vi "Condition _string.vi"(10 "Shift":string(combo)="ALL", 11 "Select Line 2":string(combo)="ST 1") -> (0 "String":string, 2 "condition":string, 3 "x .and. y?":bool)   [LabVIEW 2017]
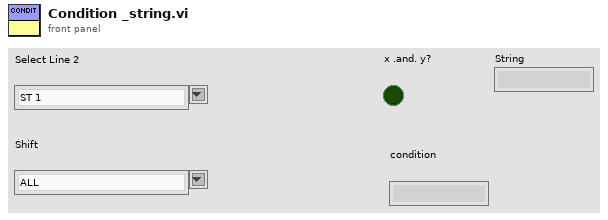
[diagram p1: front panel]
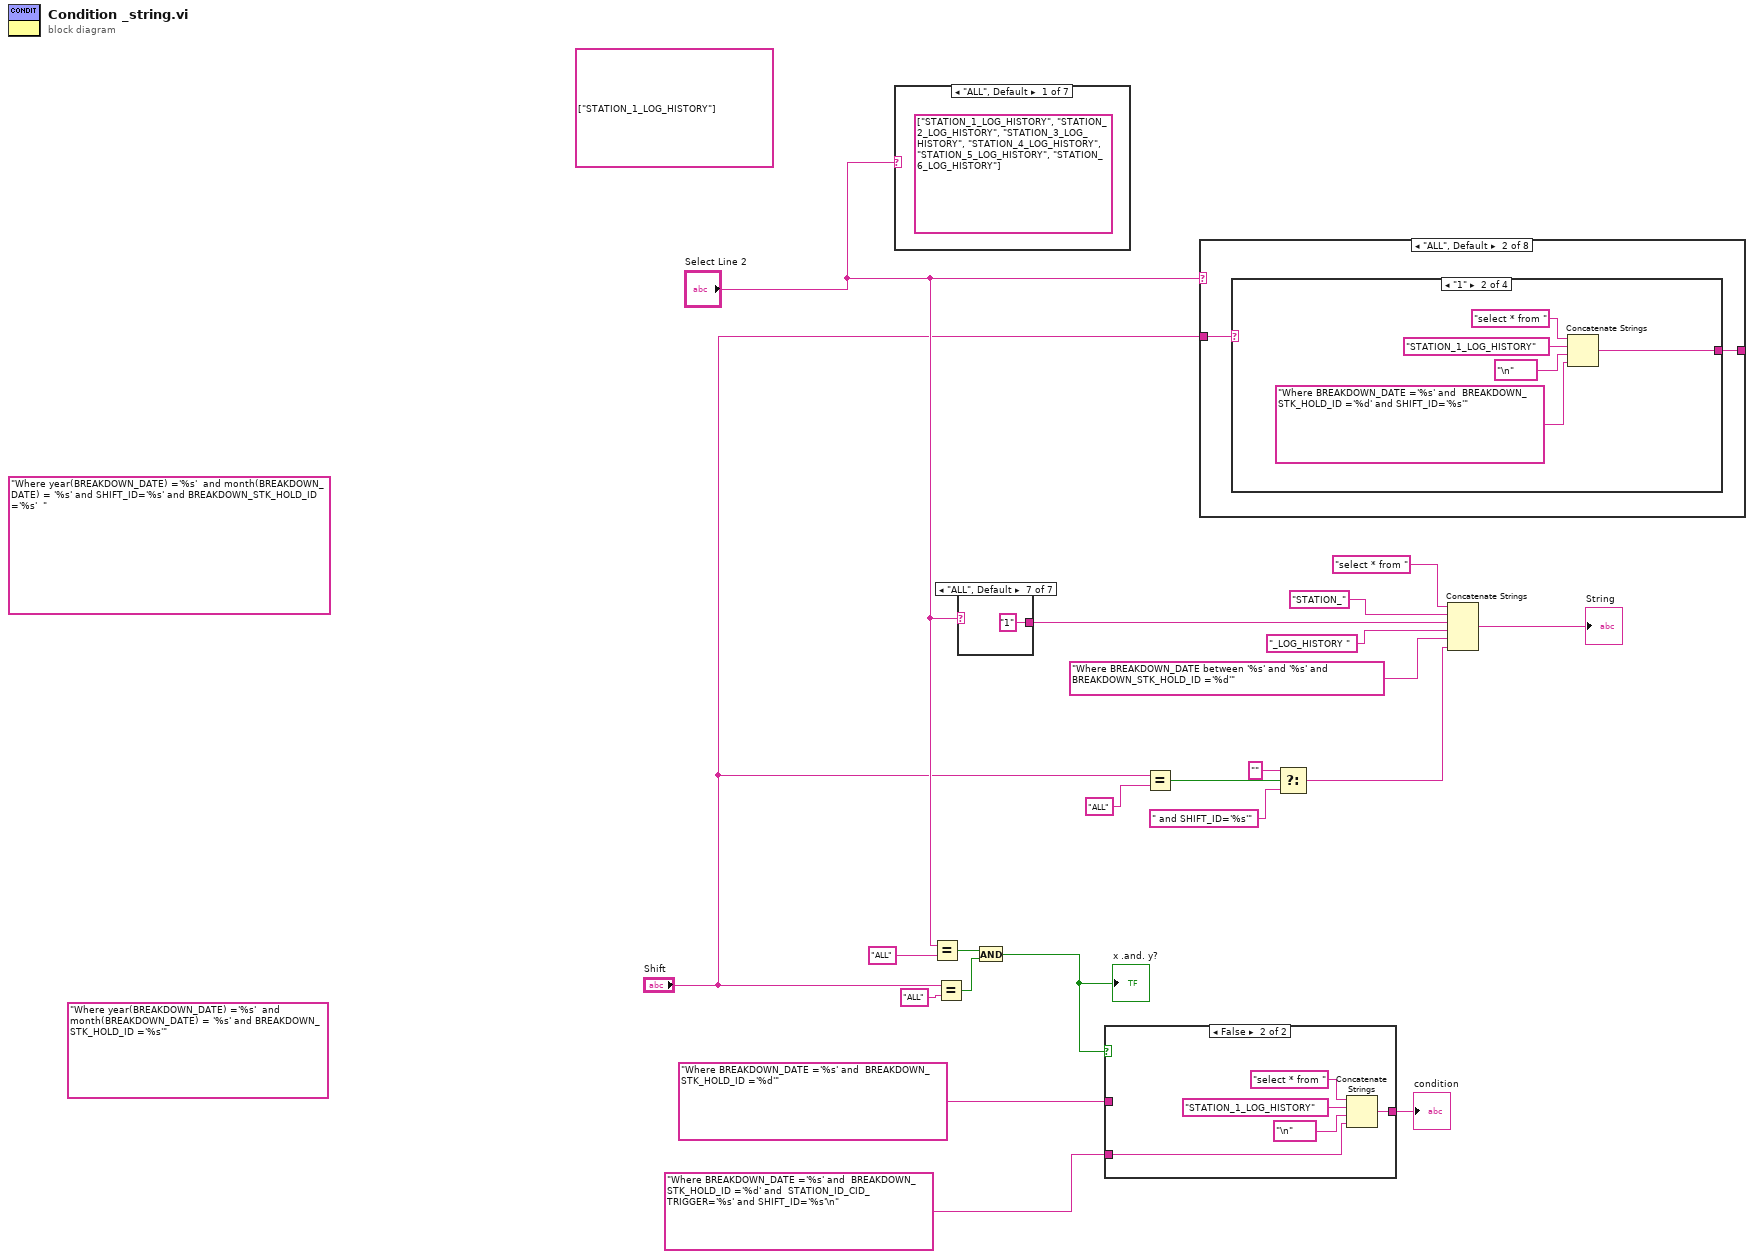
[diagram p0: block diagram]
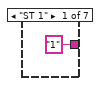
[diagram p2: hidden frame]
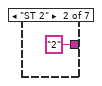
[diagram p3: hidden frame]
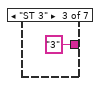
[diagram p4: hidden frame]
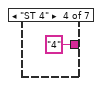
[diagram p5: hidden frame]
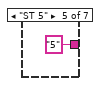
[diagram p6: hidden frame]
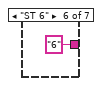
[diagram p7: hidden frame]
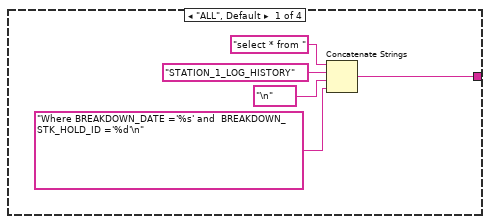
[diagram p9: hidden frame]
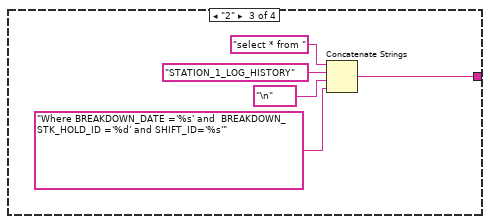
[diagram p10: hidden frame]
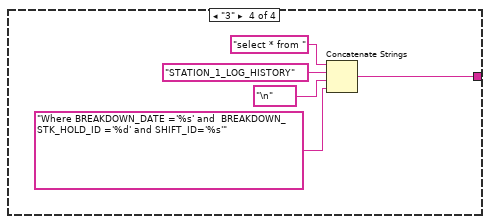
[diagram p11: hidden frame]
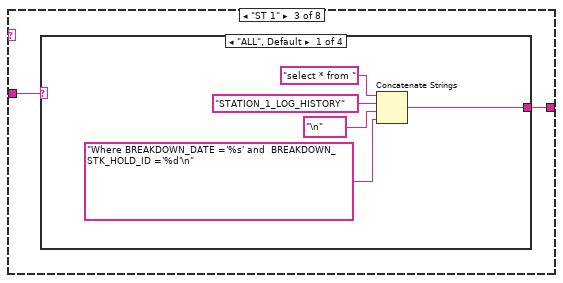
[diagram p12: hidden frame]
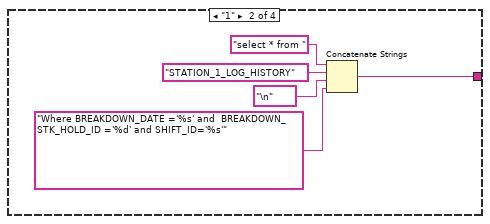
[diagram p13: hidden frame]
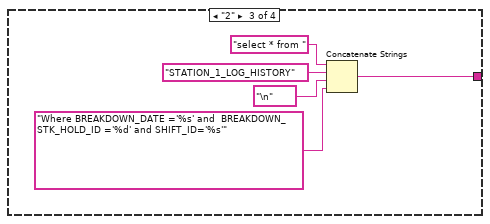
[diagram p14: hidden frame]
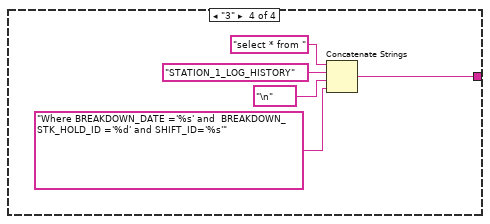
[diagram p15: hidden frame]
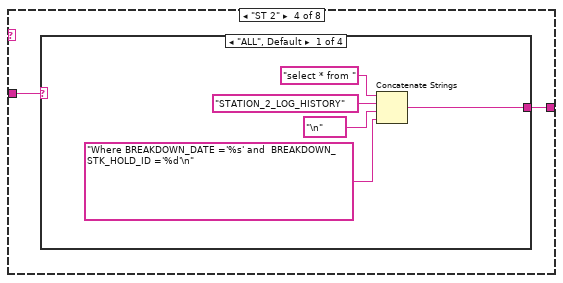
[diagram p16: hidden frame]
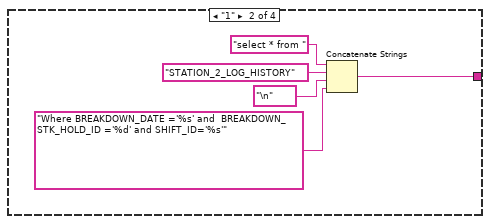
[diagram p17: hidden frame]
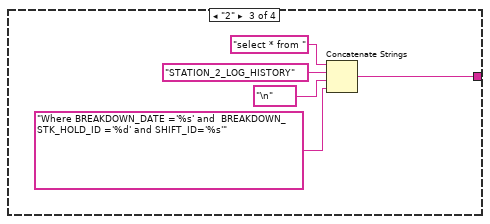
[diagram p18: hidden frame]
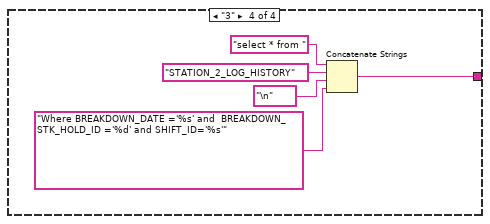
[diagram p19: hidden frame]
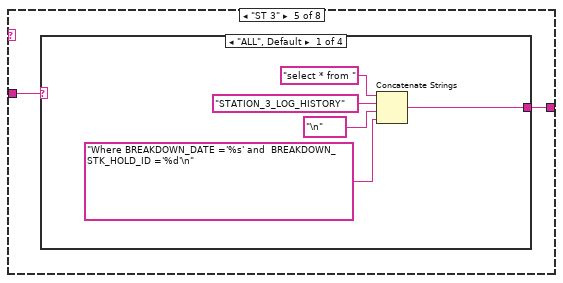
[diagram p20: hidden frame]
diagram:
  (unwired) string[] ["STATION_1_LOG_HISTORY"]
  (unwired) "Where year(BREAKDOWN_DATE) ='%s'  and month(BREAKDOWN_DATE) = '%s' and BREAKDOWN_STK_HOLD_ID ='%s'" ("condition")
  (unwired) "Where year(BREAKDOWN_DATE) ='%s'  and month(BREAKDOWN_DATE) = '%s' and SHIFT_ID='%s' and BREAKDOWN_STK_HOLD_ID ='%s'  " ("condition")
  n1 = case shown="\"ALL\", Default" "Select Line 2" {
    frame "ALL", Default {
      (unwired) string[] ["STATION_1_LOG_HISTORY", "STATION_2_LOG_HISTORY", "STATION_3_LOG_HISTORY", "STATION_4_LOG_HISTORY", "STATION_5_LOG_HISTORY", "STATION_6_LOG_HISTORY"]
    }
    frame "STATION 1" {
      (unwired) "STATION_1_LOG_HISTORY"
    }
    frame "STATION 2" {
      (unwired) string[] ["STATION_2_LOG_HISTORY"]
    }
    frame "STATION 3" {
      (unwired) string[] ["STATION_3_LOG_HISTORY"]
    }
    frame "STATION 4" {
      (unwired) string[] ["STATION_4_LOG_HISTORY"]
    }
    frame "STATION 5" {
      (unwired) string[] ["STATION_5_LOG_HISTORY"]
    }
    frame "STATION 6" {
      (unwired) string[] ["STATION_6_LOG_HISTORY"]
    }
  }
  n2 = Equal?(x="Select Line 2", y="ALL") -> (x = y?=w19:bool)
  n3 = Equal?(x="Shift", y="ALL") -> (x = y?=w18:bool)
  n4 = case shown="\"ALL\", Default" "Select Line 2" {
    tunnel: ["1" "2" "3" "4" "5" "6" "1"] -> w3
    frame "ST 1" {
    }
    frame "ST 2" {
    }
    frame "ST 3" {
    }
    frame "ST 4" {
    }
    frame "ST 5" {
    }
    frame "ST 6" {
    }
    frame "ALL", Default {
    }
  }
  n5 = And(x=w19, y=w18) -> (x .and. y?=w17:bool)
  "x .and. y?" <- w17
  n6 = case shown="False" w17 {
    tunnel: "Where BREAKDOWN_DATE ='%s' and  BREAKDOWN_STK_HOLD_ID ='%d' and  STATION_ID_CID_TRIGGER='%s' and SHIFT_ID='%s'\n" ("condition") -> [_ w35]
    tunnel: "Where BREAKDOWN_DATE ='%s' and  BREAKDOWN_STK_HOLD_ID ='%d'" ("condition") -> [w30 _]
    tunnel: [w29 w34] -> w14
    frame True {
      n7 = Concatenate Strings("select * from " ("string"), "STATION_1_LOG_HISTORY" ("table"), "\n" ("string"), w30) -> (w29:string)
    }
    frame False {
      n8 = Concatenate Strings("select * from " ("string"), "STATION_1_LOG_HISTORY" ("table"), "\n" ("string"), w35) -> (w34:string)
    }
  }
  "condition" <- w14
  n9 = Equal?(x="Shift", y="ALL" ("condition")) -> (x = y?=w8:bool)
  n10 = case shown="\"ALL\", Default" "Select Line 2" {
    tunnel: "Shift" -> [_ w40 w62 w84 w106 w128 w150 w172]
    tunnel: [_ w39 w61 w83 w105 w127 w149 w171] -> _
    frame "False" {
    }
    frame "ALL", Default {
      n11 = case shown="\"1\"" w40 {
        tunnel: [w41 w46 w51 w56] -> w39
        frame "ALL", Default {
          n12 = Concatenate Strings("select * from " ("string"), "STATION_1_LOG_HISTORY" ("table"), "\n" ("string"), "Where BREAKDOWN_DATE ='%s' and  BREAKDOWN_STK_HOLD_ID ='%d'\n" ("condition")) -> (w41:string)
        }
        frame "1" {
          n13 = Concatenate Strings("select * from " ("string"), "STATION_1_LOG_HISTORY" ("table"), "\n" ("string"), "Where BREAKDOWN_DATE ='%s' and  BREAKDOWN_STK_HOLD_ID ='%d' and SHIFT_ID='%s'" ("condition")) -> (w46:string)
        }
        frame "2" {
          n14 = Concatenate Strings("select * from " ("string"), "STATION_1_LOG_HISTORY" ("table"), "\n" ("string"), "Where BREAKDOWN_DATE ='%s' and  BREAKDOWN_STK_HOLD_ID ='%d' and SHIFT_ID='%s'" ("condition")) -> (w51:string)
        }
        frame "3" {
          n15 = Concatenate Strings("select * from " ("string"), "STATION_1_LOG_HISTORY" ("table"), "\n" ("string"), "Where BREAKDOWN_DATE ='%s' and  BREAKDOWN_STK_HOLD_ID ='%d' and SHIFT_ID='%s'" ("condition")) -> (w56:string)
        }
      }
    }
    frame "ST 1" {
      n16 = case shown="\"ALL\", Default" w62 {
        tunnel: [w63 w68 w73 w78] -> w61
        frame "ALL", Default {
          n17 = Concatenate Strings("select * from " ("string"), "STATION_1_LOG_HISTORY" ("table"), "\n" ("string"), "Where BREAKDOWN_DATE ='%s' and  BREAKDOWN_STK_HOLD_ID ='%d'\n" ("condition")) -> (w63:string)
        }
        frame "1" {
          n18 = Concatenate Strings("select * from " ("string"), "STATION_1_LOG_HISTORY" ("table"), "\n" ("string"), "Where BREAKDOWN_DATE ='%s' and  BREAKDOWN_STK_HOLD_ID ='%d' and SHIFT_ID='%s'" ("condition")) -> (w68:string)
        }
        frame "2" {
          n19 = Concatenate Strings("select * from " ("string"), "STATION_1_LOG_HISTORY" ("table"), "\n" ("string"), "Where BREAKDOWN_DATE ='%s' and  BREAKDOWN_STK_HOLD_ID ='%d' and SHIFT_ID='%s'" ("condition")) -> (w73:string)
        }
        frame "3" {
          n20 = Concatenate Strings("select * from " ("string"), "STATION_1_LOG_HISTORY" ("table"), "\n" ("string"), "Where BREAKDOWN_DATE ='%s' and  BREAKDOWN_STK_HOLD_ID ='%d' and SHIFT_ID='%s'" ("condition")) -> (w78:string)
        }
      }
    }
    frame "ST 2" {
      n21 = case shown="\"ALL\", Default" w84 {
        tunnel: [w85 w90 w95 w100] -> w83
        frame "ALL", Default {
          n22 = Concatenate Strings("select * from " ("string"), "STATION_2_LOG_HISTORY" ("table"), "\n" ("string"), "Where BREAKDOWN_DATE ='%s' and  BREAKDOWN_STK_HOLD_ID ='%d'\n" ("condition")) -> (w85:string)
        }
        frame "1" {
          n23 = Concatenate Strings("select * from " ("string"), "STATION_2_LOG_HISTORY" ("table"), "\n" ("string"), "Where BREAKDOWN_DATE ='%s' and  BREAKDOWN_STK_HOLD_ID ='%d' and SHIFT_ID='%s'" ("condition")) -> (w90:string)
        }
        frame "2" {
          n24 = Concatenate Strings("select * from " ("string"), "STATION_2_LOG_HISTORY" ("table"), "\n" ("string"), "Where BREAKDOWN_DATE ='%s' and  BREAKDOWN_STK_HOLD_ID ='%d' and SHIFT_ID='%s'" ("condition")) -> (w95:string)
        }
        frame "3" {
          n25 = Concatenate Strings("select * from " ("string"), "STATION_2_LOG_HISTORY" ("table"), "\n" ("string"), "Where BREAKDOWN_DATE ='%s' and  BREAKDOWN_STK_HOLD_ID ='%d' and SHIFT_ID='%s'" ("condition")) -> (w100:string)
        }
      }
    }
    frame "ST 3" {
      n26 = case shown="\"ALL\", Default" w106 {
        tunnel: [w107 w112 w117 w122] -> w105
        frame "ALL", Default {
          n27 = Concatenate Strings("select * from " ("string"), "STATION_3_LOG_HISTORY" ("table"), "\n" ("string"), "Where BREAKDOWN_DATE ='%s' and  BREAKDOWN_STK_HOLD_ID ='%d'\n" ("condition")) -> (w107:string)
        }
        frame "1" {
          n28 = Concatenate Strings("select * from " ("string"), "STATION_3_LOG_HISTORY" ("table"), "\n" ("string"), "Where BREAKDOWN_DATE ='%s' and  BREAKDOWN_STK_HOLD_ID ='%d' and SHIFT_ID='%s'" ("condition")) -> (w112:string)
        }
        frame "2" {
          n29 = Concatenate Strings("select * from " ("string"), "STATION_3_LOG_HISTORY" ("table"), "\n" ("string"), "Where BREAKDOWN_DATE ='%s' and  BREAKDOWN_STK_HOLD_ID ='%d' and SHIFT_ID='%s'" ("condition")) -> (w117:string)
        }
        frame "3" {
          n30 = Concatenate Strings("select * from " ("string"), "STATION_3_LOG_HISTORY" ("table"), "\n" ("string"), "Where BREAKDOWN_DATE ='%s' and  BREAKDOWN_STK_HOLD_ID ='%d' and SHIFT_ID='%s'" ("condition")) -> (w122:string)
        }
      }
    }
    frame "ST 4" {
      n31 = case shown="\"ALL\", Default" w128 {
        tunnel: [w129 w134 w139 w144] -> w127
        frame "ALL", Default {
          n32 = Concatenate Strings("select * from " ("string"), "STATION_4_LOG_HISTORY" ("table"), "\n" ("string"), "Where BREAKDOWN_DATE ='%s' and  BREAKDOWN_STK_HOLD_ID ='%d'\n" ("condition")) -> (w129:string)
        }
        frame "1" {
          n33 = Concatenate Strings("select * from " ("string"), "STATION_4_LOG_HISTORY" ("table"), "\n" ("string"), "Where BREAKDOWN_DATE ='%s' and  BREAKDOWN_STK_HOLD_ID ='%d' and SHIFT_ID='%s'" ("condition")) -> (w134:string)
        }
        frame "2" {
          n34 = Concatenate Strings("select * from " ("string"), "STATION_4_LOG_HISTORY" ("table"), "\n" ("string"), "Where BREAKDOWN_DATE ='%s' and  BREAKDOWN_STK_HOLD_ID ='%d' and SHIFT_ID='%s'" ("condition")) -> (w139:string)
        }
        frame "3" {
          n35 = Concatenate Strings("select * from " ("string"), "STATION_4_LOG_HISTORY" ("table"), "\n" ("string"), "Where BREAKDOWN_DATE ='%s' and  BREAKDOWN_STK_HOLD_ID ='%d' and SHIFT_ID='%s'" ("condition")) -> (w144:string)
        }
      }
    }
    frame "ST 5" {
      n36 = case shown="\"3\"" w150 {
        tunnel: [w151 w156 w161 w166] -> w149
        frame "ALL", Default {
          n37 = Concatenate Strings("select * from " ("string"), "STATION_5_LOG_HISTORY" ("table"), "\n" ("string"), "Where BREAKDOWN_DATE ='%s' and  BREAKDOWN_STK_HOLD_ID ='%d'\n" ("condition")) -> (w151:string)
        }
        frame "1" {
          n38 = Concatenate Strings("select * from " ("string"), "STATION_5_LOG_HISTORY" ("table"), "\n" ("string"), "Where BREAKDOWN_DATE ='%s' and  BREAKDOWN_STK_HOLD_ID ='%d' and SHIFT_ID='%s'" ("condition")) -> (w156:string)
        }
        frame "2" {
          n39 = Concatenate Strings("select * from " ("string"), "STATION_5_LOG_HISTORY" ("table"), "\n" ("string"), "Where BREAKDOWN_DATE ='%s' and  BREAKDOWN_STK_HOLD_ID ='%d' and SHIFT_ID='%s'" ("condition")) -> (w161:string)
        }
        frame "3" {
          n40 = Concatenate Strings("select * from " ("string"), "STATION_5_LOG_HISTORY" ("table"), "\n" ("string"), "Where BREAKDOWN_DATE ='%s' and  BREAKDOWN_STK_HOLD_ID ='%d' and SHIFT_ID='%s'" ("condition")) -> (w166:string)
        }
      }
    }
    frame "ST 6" {
      n41 = case shown="\"ALL\", Default" w172 {
        tunnel: [w173 w178 w183 w188] -> w171
        frame "ALL", Default {
          n42 = Concatenate Strings("select * from " ("string"), "STATION_6_LOG_HISTORY" ("table"), "\n" ("string"), "Where BREAKDOWN_DATE ='%s' and  BREAKDOWN_STK_HOLD_ID ='%d'\n" ("condition")) -> (w173:string)
        }
        frame "1" {
          n43 = Concatenate Strings("select * from " ("string"), "STATION_6_LOG_HISTORY" ("table"), "\n" ("string"), "Where BREAKDOWN_DATE ='%s' and  BREAKDOWN_STK_HOLD_ID ='%d' and SHIFT_ID='%s'" ("condition")) -> (w178:string)
        }
        frame "2" {
          n44 = Concatenate Strings("select * from " ("string"), "STATION_6_LOG_HISTORY" ("table"), "\n" ("string"), "Where BREAKDOWN_DATE ='%s' and  BREAKDOWN_STK_HOLD_ID ='%d' and SHIFT_ID='%s'" ("condition")) -> (w183:string)
        }
        frame "3" {
          n45 = Concatenate Strings("select * from " ("string"), "STATION_6_LOG_HISTORY" ("table"), "\n" ("string"), "Where BREAKDOWN_DATE ='%s' and  BREAKDOWN_STK_HOLD_ID ='%d' and SHIFT_ID='%s'" ("condition")) -> (w188:string)
        }
      }
    }
  }
  n46 = Select(t="", s=w8, f=" and SHIFT_ID='%s'" ("condition")) -> (s? t:f=w5:string)
  n47 = Concatenate Strings("select * from " ("string"), "STATION_" ("table"), w3, "_LOG_HISTORY " ("table"), "Where BREAKDOWN_DATE between '%s' and '%s' and  BREAKDOWN_STK_HOLD_ID ='%d'" ("condition"), w5) -> (→"String":string)
